vi "ProjectedDistance.vi"(6 "X Displacement":refnum<vi>, 7 "Spot Number Check":refnum<vi>, 9 "Current Spot #":refnum<vi>, 10 "Spot Checker":refnum<vi>, 11 "Y Displacement":refnum<vi>) -> (3 "Numeric":dbl)   [LabVIEW 2019]
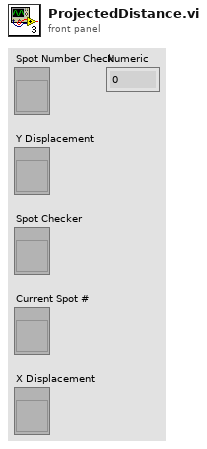
[diagram p1: front panel]
types:
  T1 = typedef "spot.ctl" = cluster{"Position":cluster{"x":dbl, "y":dbl, "z":dbl}, "Intensity":dbl, "Vortex Charge":i8, "Phase":dbl, "NA Position":cluster{"x":dbl, "y":dbl, "r":dbl}, "Line Trapping":T2, "Amplitude Correction":dbl}
  T2 = typedef "line_trapping.ctl" = cluster{"Vector":cluster{"x":dbl, "y":dbl, "z":dbl}, "Phase Gradient":dbl}
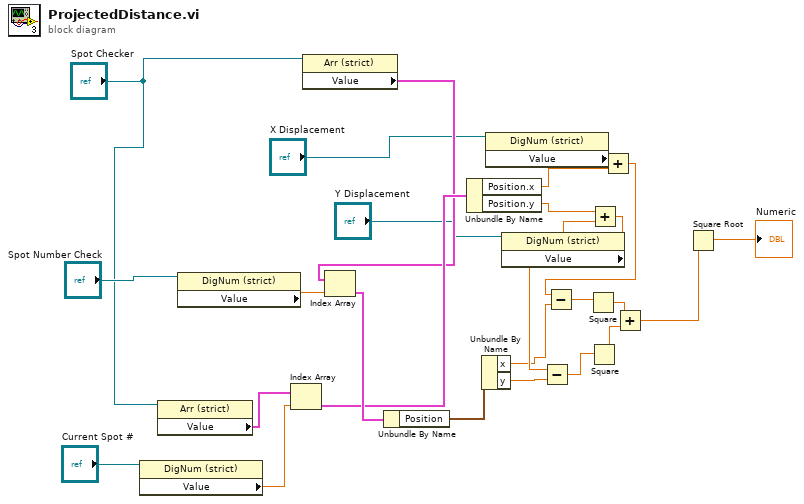
[diagram p0: block diagram]
diagram:
  n1 = property class="DigNum (strict)"(reference="Current Spot #") -> ("Value"=w17:dbl)  [unwired: 1 in, 2 out]
  n2 = property class="Arr (strict)"(reference="Spot Checker") -> ("Value"=w16:T1[])  [unwired: 1 in, 2 out]
  n3 = property class="DigNum (strict)"(reference="Spot Number Check") -> ("Value"=w14:dbl)  [unwired: 1 in, 2 out]
  n4 = Index Array(array=w16, index=w17) -> (element=w18:T1)
  n5 = property class="Arr (strict)"(reference="Spot Checker") -> ("Value"=w15:T1[])  [unwired: 1 in, 2 out]
  n6 = Index Array(array=w15, index=w14) -> (element=w19:T1)
  n7 = Unbundle By Name(w19) -> ("Position"=w13:cluster{"x":dbl, "y":dbl, "z":dbl})
  n8 = Unbundle By Name(w18) -> ("Position.x"=w21:dbl, "Position.y"=w23:dbl)
  n9 = Unbundle By Name(w13) -> ("x"=w12:dbl, "y"=w11:dbl)
  n10 = property class="DigNum (strict)"(reference="X Displacement") -> ("Value"=w22:dbl)  [unwired: 1 in, 2 out]
  n11 = property class="DigNum (strict)"(reference="Y Displacement") -> ("Value"=w24:dbl)  [unwired: 1 in, 2 out]
  n12 = Add(x=w23, y=w24) -> (x+y=w26:dbl)
  n13 = Subtract(x=w26, y=w11) -> (x-y=w9:dbl)
  n14 = Square(x=w9) -> (x^2=w7:dbl)
  n15 = Add(x=w22, y=w21) -> (x+y=w25:dbl)
  n16 = Subtract(x=w25, y=w12) -> (x-y=w10:dbl)
  n17 = Square(x=w10) -> (x^2=w8:dbl)
  n18 = Add(x=w8, y=w7) -> (x+y=w6:dbl)
  n19 = Square Root(x=w6) -> (sqrt(x)=→"Numeric":dbl)
